vi "Clean Up References and Bundle Node.vi"(6 "Total Number of Inputs":i32, 8 "error in (no error)":errorcluster, 9 "ControlReferenceConstants":refnum<vi>[](array[refnum]), 10 "Actor Input ControlTerminal":refnum<vi>, 11 "NamedBundler":refnum<vi>) -> (0 "error out":errorcluster)   [LabVIEW 2020, in "Add to Private Data.lvlib"]
uses:
  Add to Private Data.lvlib
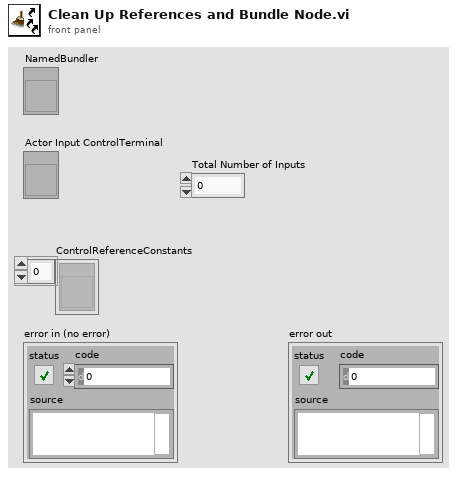
[diagram p1: front panel]
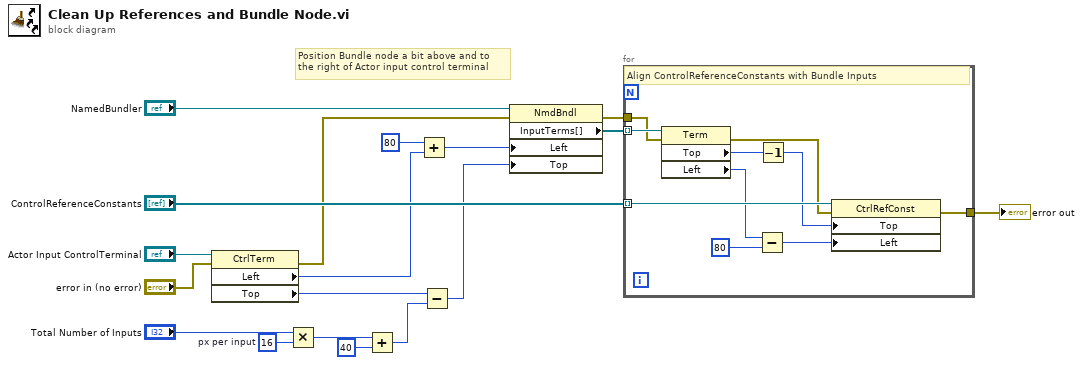
[diagram p0: block diagram]
diagram:
  w10 = 16  # px per input
  # "Position Bundle node a bit above and to\nthe right of Actor input control terminal"
  n1 = property class="CtrlTerm"(reference="Actor Input ControlTerminal", error in="error in (no error)") -> (error out=w12:errorcluster, "Left"=w5:i32, "Top"=w4:i32)  [unwired: 1 out]
  n2 = Multiply(x="Total Number of Inputs", y=w10) -> (x*y=w9:i32)
  n3 = Add(x=w9, y=40) -> (x+y=w7:i32)
  n4 = Add(x=i16 80, y=w5) -> (x+y=w15:i32)
  n5 = Subtract(x=w4, y=w7) -> (x-y=w6:i32)
  n6 = property class="NmdBndl"(reference="NamedBundler", error in=w12, "Left"=w15, "Top"=w6) -> (error out=w3:errorcluster, "InputTerms[]"=w1:refnum<vi>[])  [unwired: 1 out]
  n7 = for {
    tunnel: w1 -> [w28] mode=indexing
    tunnel: "ControlReferenceConstants" -> [w27] mode=indexing
    tunnel: w3 -> [w21]
    tunnel: [w19] -> w2
    # "Align ControlReferenceConstants with Bundle Inputs"
    n8 = property class="Term"(reference=w28, error in=w21) -> (error out=w20:errorcluster, "Top"=w26:i32, "Left"=w25:i32)  [unwired: 1 out]
    n9 = Subtract(x=w25, y=80) -> (x-y=w23:i32)
    n10 = Decrement(x=w26) -> (x-1=w22:i32)
    n11 = property class="CtrlRefConst"(reference=w27, error in=w20, "Top"=w22, "Left"=w23) -> (error out=w19:errorcluster)  [unwired: 1 out]
  }
  "error out" <- w2
